vi "SVL RMS Level (1 Ch).vi"(6 "restart averaging (F)":bool, 8 "error in (no error)":errorcluster, 11 "scaled signal [EU]":waveform(dbl)) -> (0 "error out":errorcluster, 2 "unit label":string, 3 "RMS level [EU rms]":dbl=nan format="%.2f")   [LabVIEW 2017, in "SoundVib_VibrationLevel.lvlib"]
doc: "Computes the root-mean-square (RMS) level of <B>scaled signal [EU]</B> or <B>even-angle signal [EU]</B>. <B>Scaled signal [EU]</B> should have a zero DC component. You can attenuate the DC component with hardware AC-coupling filters and with software high-pass filters. Wire data to the <B>scaled signal [EU]</B> input to determine the polymorphic instance to use or manually select the instance."
uses:
  <vilib>/addons/Sound and Vibration/svt_Level/SoundVib_VibrationLevel.lvlib
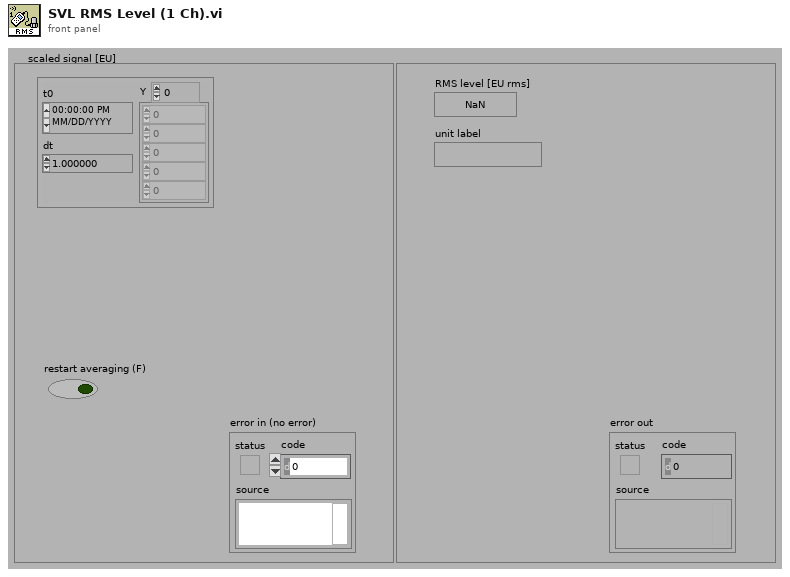
[diagram p1: front panel]
types:
  T1 = enum16{"RMS", "Running RMS", "Exp avg  ", "Dec exp avg ", "Peak", "Crest"}
  T2 = enum16{"Reset filter", "Restart averaging", "Continue processing"}
  T3 = typedef "svc_Channel Info.ctl" = cluster{"sensor sensitivity":dbl, "engineering units":T4, "dB reference":dbl, "custom label":string, "weighting filter":T5, "pregain":dbl}
  T4 = typedef "svc_Engineering Units Text Ring.ctl" = u16
  T5 = typedef "svc_Weighting Filter Text Ring.ctl" = u16
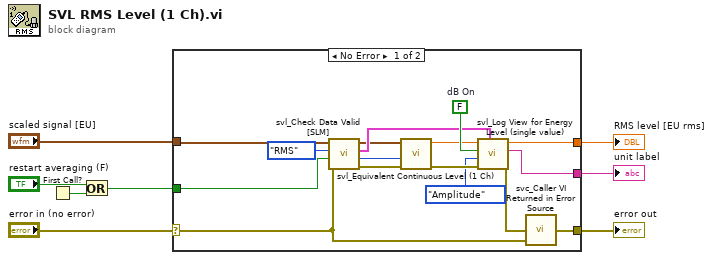
[diagram p0: block diagram]
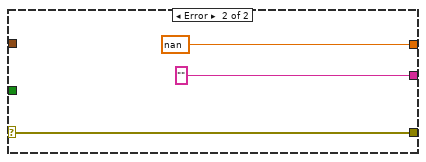
[diagram p2: hidden frame]
diagram:
  n1 = First Call?() -> (First Call?: T/F=w4:bool)
  n2 = Or(x="restart averaging (F)", y=w4) -> (x .or. y?=w2:bool)
  n3 = case shown="No Error" "error in (no error)" {
    selector: "error in (no error)" -> [w9 w27]
    tunnel: [w17 w27] -> w8
    tunnel: [w23 nan ("energy level [EU^2 rms]")] -> w7
    tunnel: [w22 "" ("unit label")] -> w6
    tunnel: "scaled signal [EU]" -> [w12 _]
    tunnel: w2 -> [w15 _]
    frame No Error {
      w20 = FALSE  # dB On
      n4 = call <vilib>:"svl_Check Data Valid [SLM].vi"("error in (no error)"=w9, "restart averaging (F)"=w15, "Level Analysis"=T1."RMS", "scaled signal [EU]"=w12) -> ("error out"=w16:errorcluster, "processing state"=w14:T2, "channel info"=w11:T3, "dup scaled signal [EU]"=w10:waveform(dbl))  [unwired: 4 in]
      n5 = call <vilib>:"svl_Equivalent Continuous Level (1 Ch).vi"("error in (no error)"=w16, "processing state"=w14, "scaledSignal"=w10) -> ("error out"=w21:errorcluster, "equivalent continuous level [EU^2 rms]"=w19:dbl)  [unwired: 7 in]
      n6 = call <vilib>:"svl_Log View for Energy Level (single value).vi"("channel info"=w11, "error in (no error)"=w21, "view mode"=enum16{"Power", "Amplitude"}."Amplitude", "dB On (T)"=w20, "energy level [EU^2 rms]"=w19) -> ("error out"=w24:errorcluster, "unit label"=w22:string, "energy level [EU^2 rms]"=w23:dbl)  [unwired: 4 in]
      n7 = call <vilib>:"svc_Caller VI Returned in Error Source.vi"("warning input to caller"=w9, "error in (no error)"=w24) -> ("error out"=w17:errorcluster)  [unwired: 3 in]
    }
    frame Error {
    }
  }
  "RMS level [EU rms]" <- w7
  "unit label" <- w6
  "error out" <- w8
